vi "FXP_C_xhat.vi"(8 "NS":u8=9) -> (2 "y_hat":fxp<+/-,32,16>)   [LabVIEW 2017]
doc: "Given an input array X and a reference to a memory item, comput the dot product,\neg K.*X. X can be a vector up to length = 9.\n\nND is the size of the vectors.\n\n\nTHIS VI IS DIFFERENT FROM \"SGL_K2_times_xd\" by different sizes allowed."
uses:
  <vilib>/Platform/TimedLoop/XDataNode/timing_clust.ctl
  <vilib>/Platform/TimedLoop/XDataNode/nitl_modes.ctl
  <vilib>/Platform/TimedLoop/XDataNode/wakeup.ctl
  fixed-point-ss/typeDefs/x_vec_bram.ctl
  fixed-point-ss/typeDefs/Cz_zaxis_bram.ctl
  <vilib>/rvi/IPIntegrationNode/IPINode_Typedef/niFpgaIPINodeSupportedFamilies.ctl
  <vilib>/rvi/Emulation/niFpgaSctlEmulationGetInTimedLoop.vi
  <vilib>/rvi/Emulation/niFpgaEmulationReportErrorSimple.vi
  <vilib>/rvi/Emulation/niFpgaGetClockAttributes.vi
  <vilib>/rvi/Emulation/niFpgaCriticalErrorInLSC.vi
  <vilib>/rvi/DataTransferAndStorage/Container/Common/niFpgaContainerExecOnDevCompGetState.vi
  <vilib>/rvi/Emulation/niFpgaEmulationIsFPGAContextNoSignature.vi
  <vilib>/rvi/DataTransferAndStorage/Container/Common/niFpgaContainerGetUniqueNameForEmu.vi
  <vilib>/rvi/Emulation/niFpgaProcessEmulError.vi
  <vilib>/rvi/errors/nirviReportUnexpectedCaseInternalError (U32).vi
  <vilib>/rvi/Memory/Memory_Emulation/niFpgaMemoryEmulationCacheClearOnFirstRun.vi
  <vilib>/rvi/Memory/Memory_Emulation/nirvimemoryEmulationManagerCache_MakeExclusive.vi
  <vilib>/rvi/Memory/Memory_Emulation/niFpgaMemoryEmulationValidateCache.vi
  <vilib>/rvi/Memory/Memory_Emulation/nirvimemoryEmulationManagerCache_InsertValue.vi
  <vilib>/Utility/error.llb/Clear Errors.vi
  <vilib>/rvi/Memory/Memory_Emulation/nirvimemoryEmulationManagerCache_ReleaseExclusive.vi
  <vilib>/rvi/Memory/Memory_Emulation/nirvimemoryEmulationManagerCache_GetValue.vi
  <vilib>/rvi/Memory/Memory_Emulation/nirvimemoryEmulationManagerCache_SetValue.vi
  <vilib>/rvi/Emulation/niFpgaSctlEmulationResourceMgr.vi
  <vilib>/rvi/IPIntegrationNode/IPINode_Utilities/niFpgaIPINodeSimCore.vi
  <vilib>/Platform/TimedLoop/XDataNode/XDataNode.xnode
  <vilib>/rvi/DataTransferAndStorage/Container/XNode/niFpgaContainer.xnode
  <vilib>/rvi/Memory/Memory_Emulation/niFpgaMemoryEmulationRefIn.vi
  <vilib>/rvi/XilinxIP/XIPIN_XNode/niFpgaXIPIN.xnode
  fixed-point-ss/dspAccumulators/MAC1/Multiply_Accumulator_D8DE52605E734182ABB00CFADECE4F1B.dll
  <vilib>/rvi/IPIntegrationNode/IPINode_Xnode/niFpgaIPINode.xnode
  <vilib>/Platform/TimedLoop/XDataNode/XDNodeRunTimeDep.lvlib
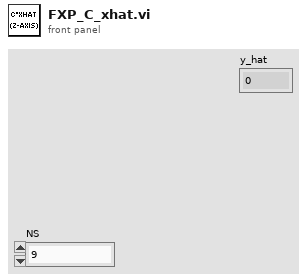
[diagram p1: front panel]
types:
  T1 = typedef "XDNodeRunTimeDep.lvlib/timing_clust.ctl" = cluster{"Expected End [f-1]":u64, "Actual End [f-1]":u64, "Finished Late? [f-1]":bool, "Expected End [i-1]":u64, "Actual End [i-1]":u64, "Finished Late? [i-1]":bool, "Expected Start [i]":u64, "Actual Start [i]":u64, "Expected Start [f]":u64, "Actual Start [f]":u64, "Source Name":string, "Structure Name":string, "Period":i64, "Deadline":i64, "Offset":i64, "Start":i64, "Priority":i32, "Timeout":i32, "Mode":T2, "Wakeup Reason":T3, "Error":errorcluster, "Source Type":string, "Secondary Source Type":string, "Global End Time":u64, "Global Start Time":u64, "Frame Duration":u64, "Iteration Duration":u64, "Assigned CPU":i32, "I/O Scan Engine Mode":u32}
  T2 = typedef "XDNodeRunTimeDep.lvlib/nitl_modes.ctl" = enum32{"No Change", "Process missed periods, maintain original phase", "Discard missed periods, maintain original phase", "Process missed periods, ignore original phase", "Discard missed periods, ignore original phase"}
  T3 = typedef "XDNodeRunTimeDep.lvlib/wakeup.ctl" = enum32{"Normal", "Aborted", "Asynchronous wakeup", "Timing source error", "Timed loop error", "Timeout"}
  T4 = typedef "Cz_zaxis_bram.ctl" = refnum<k21>
  T5 = typedef "x_vec_bram.ctl" = refnum<k21>
  T6 = typedef "niFpgaIPINodeSupportedFamilies.ctl" = cluster{"unlimited?":bool, "supported targets":string[]}
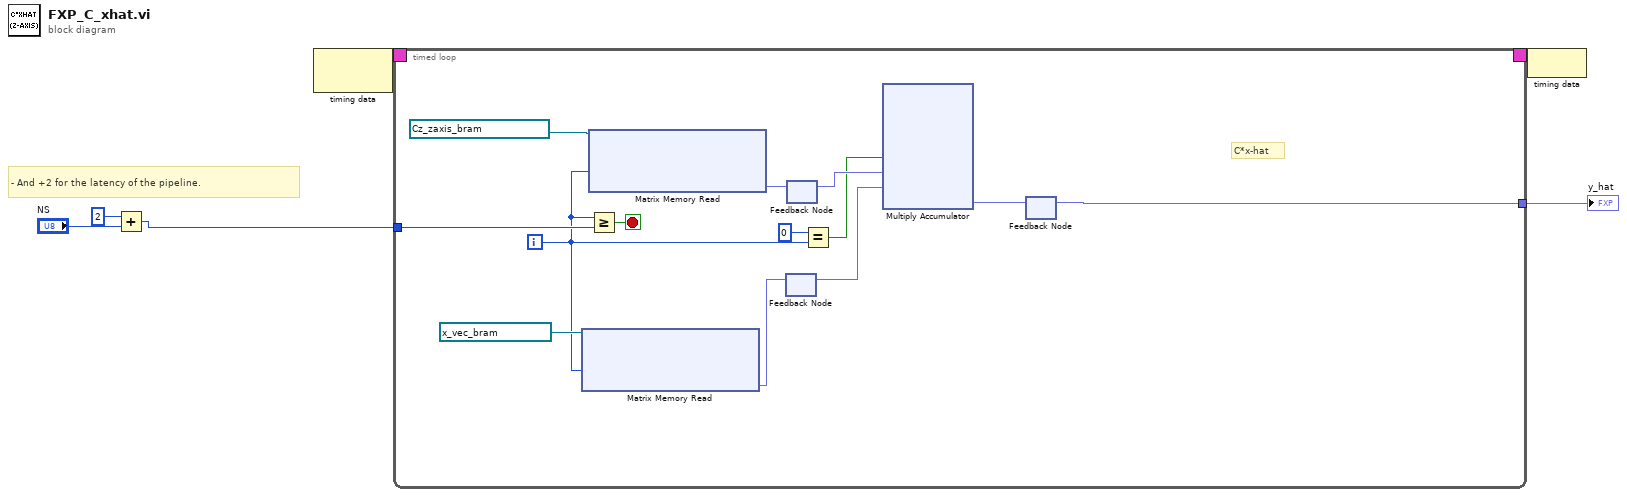
[diagram p0: block diagram]
diagram:
  # "- And +2 for the latency of the pipeline."
  n1 = Add(x=u8 2, y="NS") -> (x+y=w3:u8)
  n2 = node-c288() -> (w6:T1)  [unwired: 1 in]
  n3 = timed-loop {
    timing: w6 -> [_]
    timing-out: [_] -> w5
    tunnel: w3 -> [w18]
    tunnel: [w8] -> w1
    i -> [w11]
    stop <- w19 stop-if-true
    # "C*x-hat"
    n4 = xnode "Matrix Memory Read"("Address"=w11, "Memory In"=T5 "xk_0_2_zaxis" ("Memory")) -> ("Data"=w10:fxp<+/-,32,6>)  [unwired: 1 out]
    n5 = xnode "Matrix Memory Read"("Address"=w11, "Memory In"=T4 "C_FXP_row1_zaxis" ("Memory")) -> ("Data"=w16:fxp<+/-,32,5>)  [unwired: 1 out]
    n6 = Greater Or Equal?(x=w11, y=w18) -> (x >= y?=w19:bool)
    n7 = feedback #1() -> (w15:fxp<+/-,32,6>)  [unwired: 1 in]
    n8 = feedback-in #1(w10) -> ()
    n9 = feedback-in #2(w16) -> ()
    n10 = feedback #2() -> (w13:fxp<+/-,32,5>)  [unwired: 1 in]
    n11 = Equal?(x=0, y=w11) -> (x = y?=w9:bool)
    n12 = xnode ("Multiply Accumulator")("sclr"=w9, "a"=w13, "b"=w15) -> ("s"=w14:fxp<+/-,32,16>)  [unwired: 1 in]
    n13 = feedback #3() -> (w8:fxp<+/-,32,16>)  [unwired: 1 in]
    n14 = feedback-in #3(w14) -> ()
  }
  "y_hat" <- w1
  n15 = node-c288(w5) -> ()
